vi "Logarithm10 of SGL (2012).vi"(9 "Input Valid":bool=TRUE, 10 "Input Number (SGL)":fxp<+,32,32> format="%.0b") -> (1 "Output Valid":bool, 2 "Logarithm":fxp<+/-,34,12> format="%.26g")   [LabVIEW 2012]
doc: "<b> Latency = 9 Ticks </b>"
uses:
  <vilib>/rvi/DataTransferAndStorage/Container/Common/niFpgaContainerMetaDataKey.ctl
  <vilib>/rvi/DataTransferAndStorage/Container/Common/niFpgaContainerState.ctl
  <vilib>/rvi/DataTransferAndStorage/Container/Common/niFpgaDataTypeControl.ctl
  <vilib>/rvi/DataTransferAndStorage/Container/Common/niFpgaContainerImplementationControl.ctl
  <vilib>/rvi/DataTransferAndStorage/Container/Common/niFpgaContainerArbitrationOptionsControl.ctl
  <vilib>/rvi/DataTransferAndStorage/Container/Common/niFpgaTransferTypeControl.ctl
  <vilib>/rvi/DataTransferAndStorage/Container/Common/niFpgaContainerInitializationParameters.ctl
  <vilib>/rvi/Memory/Memory_Types/niFpgaMemoryInterfaceConfiguration.ctl
  <vilib>/rvi/FIFO/Fifo_Types/niFpgaFifoControlLogicControl.ctl
  <vilib>/rvi/Emulation/niFpgaSctlEmulationGetInTimedLoop.vi
  <vilib>/rvi/DataTransferAndStorage/Container/Common/niFpgaContainerGetUniqueNameForEmu.vi
  <vilib>/rvi/DataTransferAndStorage/Container/Common/niFpgaContainerSetEmuInfo.vi
  <vilib>/rvi/eio/common/nirviEmuReportErrorAndStop.vi
  <vilib>/rvi/DataTransferAndStorage/Container/Common/niFpgaContainerExecOnDevCompGetState.vi
  <vilib>/rvi/Memory/Memory_Emulation/niFpgaMemoryEmulationCacheClearOnFirstRun.vi
  <vilib>/rvi/Memory/Memory_Emulation/nirvimemoryEmulationManagerCache_MakeExclusive.vi
  <vilib>/rvi/Memory/Memory_Emulation/niFpgaMemoryEmulationValidateCache.vi
  <vilib>/rvi/Memory/Memory_Emulation/nirvimemoryEmulationManagerCache_ReleaseExclusive.vi
  <vilib>/rvi/Memory/Memory_Emulation/nirvimemoryEmulationManagerCache_InsertValue.vi
  <vilib>/Utility/error.llb/Clear Errors.vi
  <vilib>/rvi/Memory/Memory_Emulation/nirvimemoryEmulationManagerCache_GetValue.vi
  <vilib>/rvi/FXPMathLib/basic elements/FxpDiscreteDelay/XNode/nifxpmath_DiscreteDelay.xnode
  <vilib>/rvi/LocalResourceManager/LocalResourceManager.xnode
  <vilib>/rvi/DataTransferAndStorage/Container/XNode/niFpgaContainer.xnode
  <vilib>/rvi/Memory/Memory_Emulation/niFpgaMemoryEmulationRefIn.vi
panel:
  out "Exponent (-N)":u8
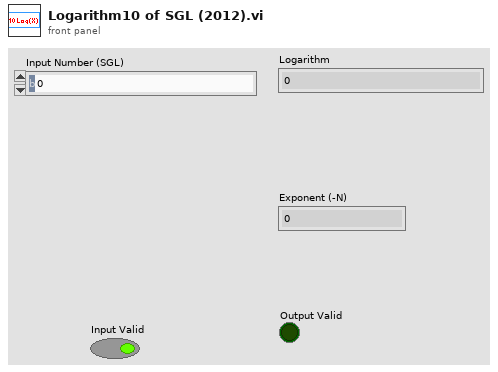
[diagram p1: front panel]
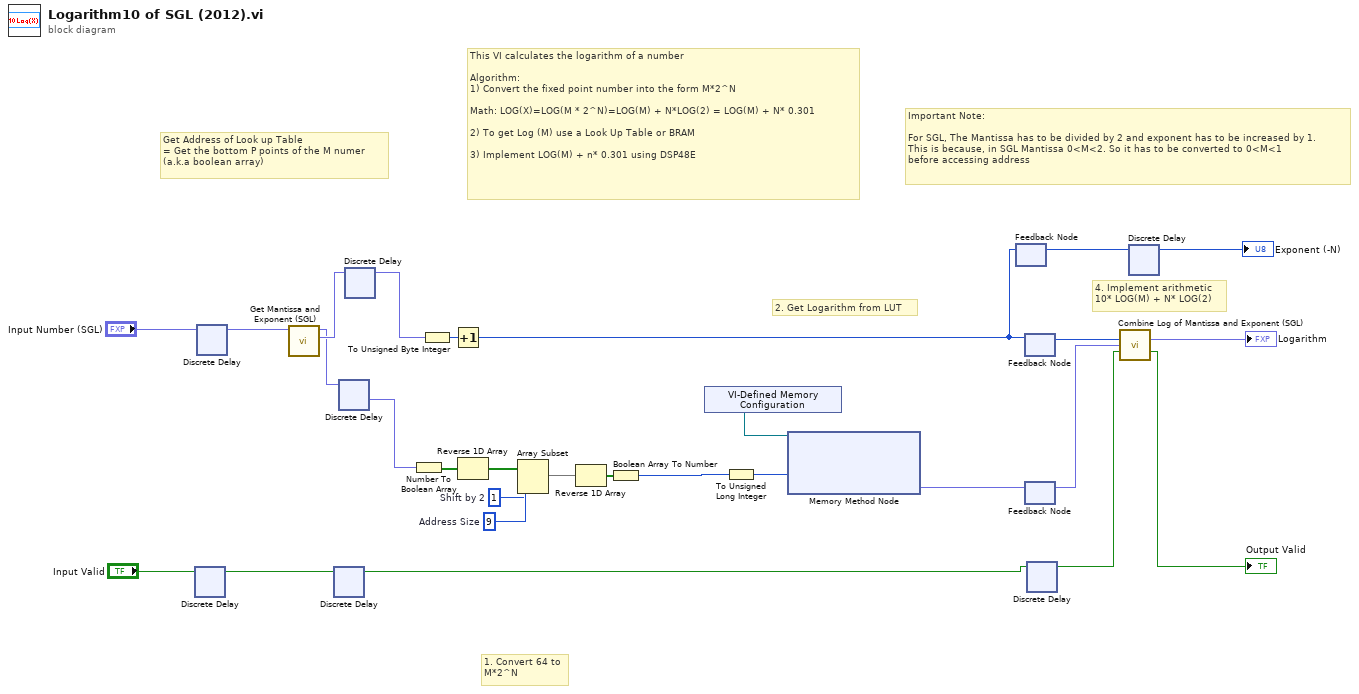
[diagram p0: block diagram]
diagram:
  w8 = 1  # Shift by 2
  w28 = 9  # Address Size
  # "Important Note:\n\nFor SGL, The Mantissa has to be divided by 2 and exponent has to be increased by 1.\nThis is because, in SGL Mantissa 0<M<2. So it has to be converted to 0<M<1\nbefore accessing address"
  # "4. Implement arithmetic\n10* LOG(M) + N* LOG(2)"
  # "2. Get Logarithm from LUT"
  # "1. Convert 64 to\nM*2^N"
  # "This VI calculates the logarithm of a number\n\nAlgorithm:\n1) Convert the fixed point number into the form M*2^N\n\nMath: LOG(X)=LOG(M * 2^N)=LOG(M) + N*LOG(2) = LOG(M) + N* 0.301 \n\n2) To get Log (M) use a Look Up Table or BRAM\n\n3) Implement LOG(M) + n* 0.301 using DSP48E"
  # "Get Address of Look up Table\n= Get the bottom P points of the M numer\n(a.k.a boolean array)"
  n1 = xnode ("Discrete Delay")("D"="Input Valid") -> ("Q"=w12:bool)
  n2 = xnode ("Discrete Delay")("D"="Input Number (SGL)") -> ("Q"=w10:fxp<+,32,32>)
  n3 = call <userlib>:"Get Mantissa and Exponent (SGL).vi"("Input"=w10) -> ("Exponent"=w14:fxp<+/-,8,8>, "FXP Part"=w13:fxp<+/-,25,2>)  [unwired: 8 in, 1 out]
  n4 = xnode ("Discrete Delay")("D"=w12) -> ("Q"=w1:bool)
  n5 = xnode ("Discrete Delay")("D"=w13) -> ("Q"=w5:fxp<+/-,25,2>)
  n6 = xnode ("Discrete Delay")("D"=w14) -> ("Q"=w4:fxp<+/-,8,8>)
  n7 = Number To Boolean Array(number=w5) -> (Boolean array=w27:bool[])
  n8 = To Unsigned Byte Integer(number=w4) -> (unsigned 8bit integer=w9:u8)
  n9 = Increment(x=w9) -> (x+1=w6:u8)
  n10 = Reverse 1D Array(array=w27) -> (reversed array=w26:bool[])
  n11 = Array Subset(array=w26, index=w8, length=w28) -> (w25:bool[])
  n12 = Reverse 1D Array(array=w25) -> (reversed array=w24:bool[])
  n13 = Boolean Array To Number(Boolean array=w24) -> (number=w23:u16)
  n14 = xnode "VI-Defined Memory Configuration"() -> ("Memory Out"=w2:refnum<k21>)
  n15 = To Unsigned Long Integer(number=w23) -> (unsigned 32bit integer=w3:u32)
  n16 = xnode ("Memory Method Node")("Address"=w3, "Memory In"=w2) -> ("Data"=w7:fxp<+/-,18,8>)  [unwired: 1 out]
  n17 = feedback #1() -> (w16:u8)  [unwired: 1 in]
  n18 = feedback-in #1(w6) -> ()
  n19 = feedback #2() -> (w20:u8)  [unwired: 1 in]
  n20 = feedback-in #2(w6) -> ()
  n21 = feedback #3() -> (w21:fxp<+/-,18,8>)  [unwired: 1 in]
  n22 = feedback-in #3(w7) -> ()
  n23 = xnode "Discrete Delay"("D"=w1) -> ("Q"=w18:bool)
  n24 = call <userlib>:"Combine Log of Mantissa and Exponent (SGL).vi"("Exponent of 2"=w20, "10Log (Mantissa)"=w21, "Input Valid"=w18) -> ("Logarithm"=→"Logarithm":fxp<+/-,34,12>, "Output Valid"=→"Output Valid":bool)  [unwired: 11 in]
  n25 = xnode ("Discrete Delay")("D"=w16) -> ("Q"=→"Exponent (-N)":u8)
